vi "UTIL Update Moving Average.vi"(8 "Error In":errorcluster, 10 "Data In":dbl[](array[numeric]), 11 "Average Queue":refnum<queue>) -> (0 "Error Out":errorcluster, 3 "Average":dbl[](array[numeric]))   [LabVIEW 2017]
doc: "This computes a backward Moving Average, using a fixed-length Queue to hold the last N points. The algorithm is simple -- do a Lossy Enqueue, which bumps out the oldest point, use the Get Queue Status to get the Queue contents (without emptying the Queue) and return the Mean.\n\nInput:\n Average Qyeye Fixed-length Queue of Dbl\n DataPoint Dbl\n Error In\nOutput:\n Moving Average Dbl\n Error Out"
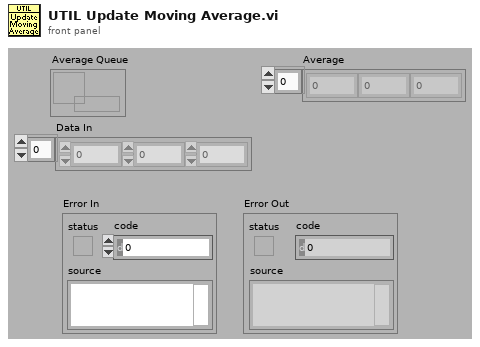
[diagram p1: front panel]
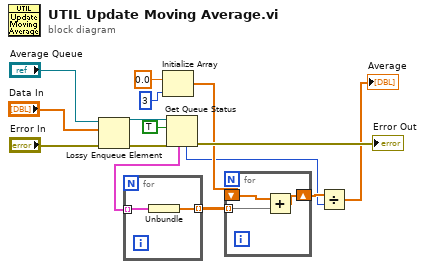
[diagram p0: block diagram]
diagram:
  n1 = Lossy Enqueue Element(queue="Average Queue", element="Data In", error in (no error)="Error In") -> (queue out=w12:refnum<queue>, error out=w13:errorcluster)  [unwired: 2 out]
  n2 = Initialize Array(0.0 ("element"), 3 ("dimension size")) -> (w4:dbl[])
  n3 = Get Queue Status(queue=w12, return elements? (F)=TRUE, error in (no error)=w13) -> (error out=→"Error Out":errorcluster, # elements in queue=w2:i32, elements=w8:cluster{dbl[]}[])  [unwired: 5 out]
  n4 = for {
    tunnel: w8 -> [w17] mode=indexing
    tunnel: [w16] -> w7 mode=indexing
    n5 = Unbundle(w17) -> (w16:dbl[])
  }
  n6 = for {
    tunnel: w7 -> [w20] mode=indexing
    shift-right: [w19] -> w3
    shift-left: w4 -> [w18]
    n7 = Add(x=w18, y=w20) -> (x+y=w19:dbl[])
  }
  n8 = Divide(x=w3, y=w2) -> (x/y=→"Average":dbl[])
